vi "Creators Creator Queue.vi"(9 "Priority?":bool, 10 "Msg Strategy":refnum<class "Msg Strategy.lvclass">, 11 "Base Event in":refnum<class "Base Event.lvclass">) -> (3 "Base Event out":refnum<class "Base Event.lvclass">)   [LabVIEW 2021, in "jettl.lvlib" / "Base Event.lvlib" / "Base Event.lvclass"]
uses:
  Base Event.lvclass
  Addresses/Addresses.lvlib
  C:/git/jettl/jettl/jettl/jettl/jettl.lvclass
  C:/git/jettl/jettl/Merge Error Msg Strategy/Merge Error/Merge Error.lvclass
  C:/git/jettl/jettl/jettl/Event/Event.lvclass
  C:/git/jettl/jettl/jettl/Last Ack Creator Queue Msg Strategy/Last Ack Creator Queue/Last Ack Creator Queue.lvclass
  C:/git/jettl/jettl/Override Error Msg Strategy/Override Error/Override Error.lvclass
  C:/git/jettl/jettl/Set Panel State Msg Strategy/Set Panel State/Set Panel State.lvclass
  C:/git/jettl/jettl/Setup Msg Strategy/Setup/Setup.lvclass
  C:/git/jettl/jettl/Teardown Msg Strategy/Teardown/Teardown.lvclass
  C:/git/jettl/jettl/jettl/Base Event/Base Event/Base Event.lvclass
  Msg Strategy/Msg Strategy.lvclass
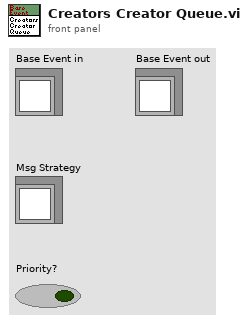
[diagram p1: front panel]
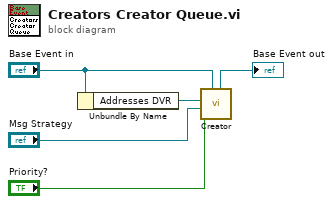
[diagram p0: block diagram]
diagram:
  n1 = Unbundle By Name("Base Event in") -> ("Addresses DVR"=w5:refnum<data-value>)
  n2 = call "Creator.vi"("jettl in"="Base Event in", "Priority?"="Priority?", "Msg Strategy"="Msg Strategy", "Addresses DVR"=w5) -> ("jettl out"=→"Base Event out":refnum<class "Base Event.lvclass">)  [unwired: 7 in]
